vi "slope_test.vi"() -> ()   [LabVIEW 2020]
uses:
  <vilib>/measure/NI_MABase.lvlib
panel:
  out "angle":dbl[](array[numeric])
  in  "butterwort filter":bool
  out "slope":dbl[](array[numeric])
  in  "end":dbl=100.0 format="%#_13g"
  out "crossings":dbl[](array[numeric])
  out "peak locations":dbl[](array[numeric])
  out "mean of peaks":dbl format="%0.2f"
  in  "amplitude":dbl=1.0 format="%0.2p"
  in  "frequency":dbl=10.0 format="%0.2p"
  out "XY Graph":cluster{"Array":dbl[], "Amplitudes":dbl[]}[](graph)
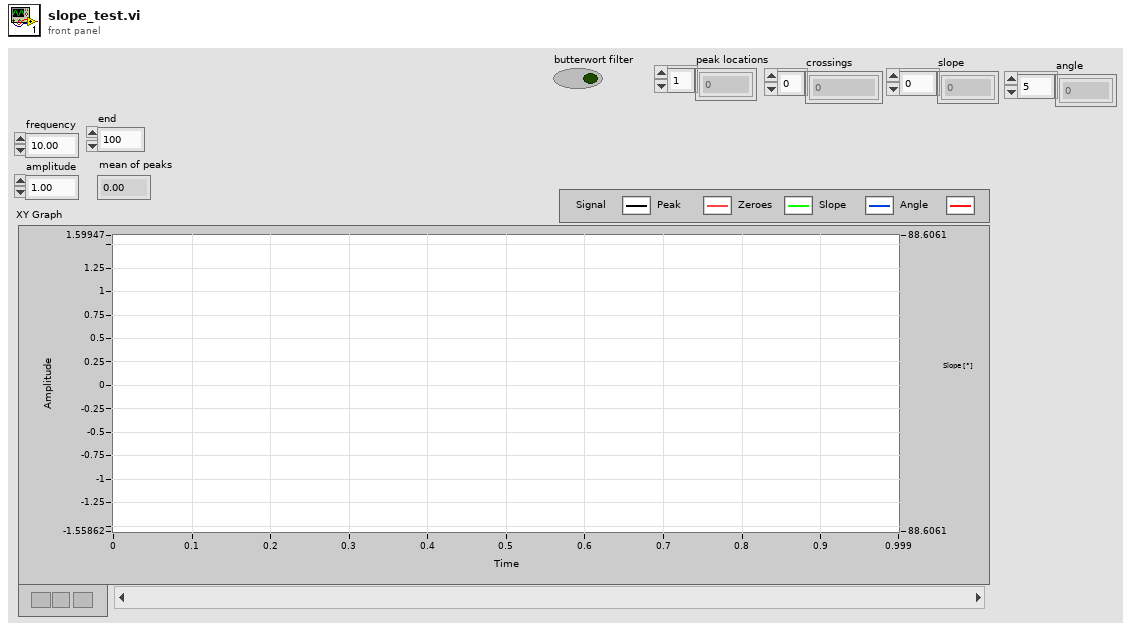
[diagram p1: front panel]
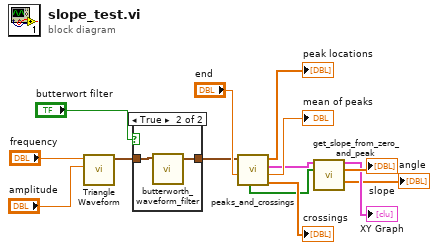
[diagram p0: block diagram]
diagram:
  n1 = call <vilib>:"Triangle Waveform.vi"("amplitude"="amplitude", "frequency"="frequency") -> ("signal out"=w7:waveform(dbl))  [unwired: 8 in, 1 out]
  n2 = case shown="True" "butterwort filter" {
    tunnel: [w15 w17] -> w8
    tunnel: w7 -> [w15 w16]
    frame False {
    }
    frame True {
      n3 = call "butterworth_waveform_filter.vi"("input"=w16) -> ("filtered"=w17:waveform(dbl))  [unwired: 4 in, 1 out]
    }
  }
  n4 = call "peaks_and_crossings.vi"("end"="end", "waveform"=w8) -> ("crossings"=→"crossings":dbl[], "mean of peaks"=→"mean of peaks":dbl, "all in array"=w4:cluster{dbl[], "Amplitudes":dbl[]}[], "peak locations"=→"peak locations":dbl[], "minus-plus crossing?"=w5:bool[])  [unwired: 3 in, 2 out]
  n5 = call "get_slope_from_zero_and_peak.vi"("All in array"=w4, "minus-plus crossing?"=w5) -> ("XY Graph"=→"XY Graph":cluster{"Array":dbl[], "Amplitudes":dbl[]}[], "slope"=→"slope":dbl[], "angle"=→"angle":dbl[])  [unwired: 8 in, 3 out]
